vi "Get Access Mode.vi"(8 "error in (no error)":errorcluster, 11 "Process In":refnum<class "Process.lvclass">) -> (0 "error out":errorcluster, 2 "Access Mode":T1, 3 "Process Out":refnum<class "Process.lvclass">)   [LabVIEW 2020, in "Process.lvclass"]
doc: "Get the recommended access mode for accessing the class attributes. Request means that a request should be made to the running process and Read means that the data should be read directly from the attributes."
uses:
  Process.lvclass
  TypeDefs/Access Mode.ctl
  Process.lvclass/Process.ctl
  <vilib>/Utility/error.llb/Clear Errors.vi
  <vilib>/Utility/error.llb/Error Cluster From Error Code.vi
  <vilib>/ErrorRing/Error Ring.xnode
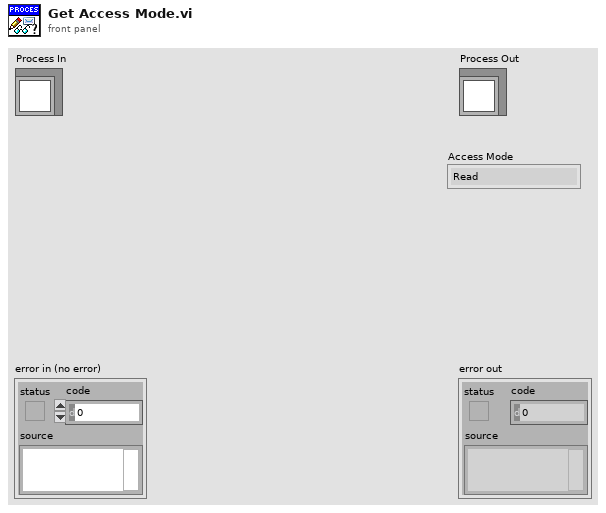
[diagram p1: front panel]
types:
  T1 = typedef "Process.lvclass/Access Mode.ctl" = enum16{"Read", "Request"}
  T2 = typedef "Process.lvclass/Lifecycle State.ctl" = enum16{"Uninitialized", "Initialized", "Started", "Running", "Stopped", "Finished"}
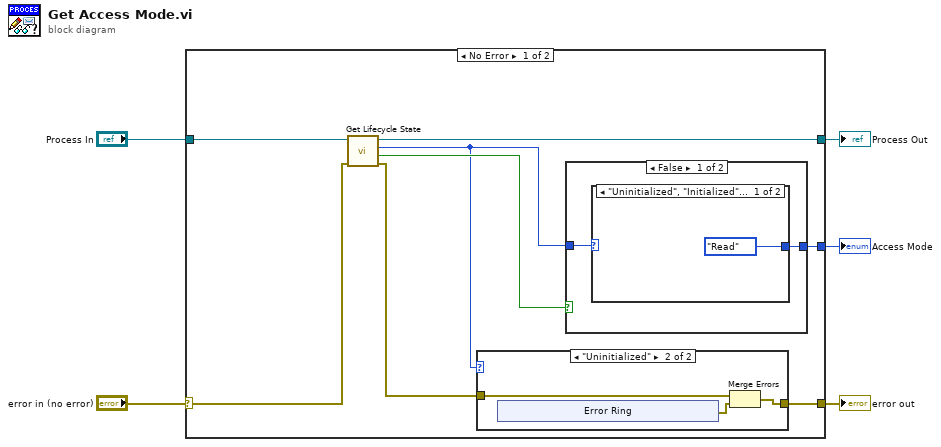
[diagram p0: block diagram]
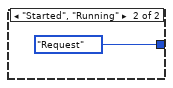
[diagram p3: hidden frame]
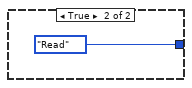
[diagram p4: hidden frame]
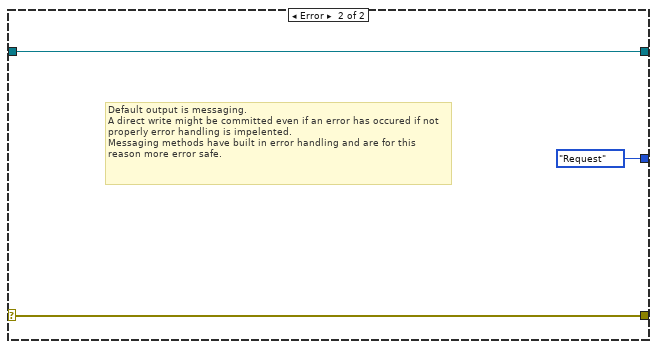
[diagram p5: hidden frame]
diagram:
  n1 = case shown="No Error" "error in (no error)" {
    selector: "error in (no error)" -> [w11 w27]
    tunnel: "Process In" -> [w13 w29]
    tunnel: [w12 w29] -> w4
    tunnel: [w7 w27] -> w2
    tunnel: [w9 Access_Mode."Request" ("Access Mode")] -> w1
    frame No Error {
      n2 = call "Get Lifecycle State.vi"("error in (no error)"=w11, "Process In"=w13) -> ("error out"=w6:errorcluster, "In Process Loop?"=w10:bool, "Lifecycle State"=w8:T2, "Process Out"=w12:refnum<class "Process.lvclass">)  [unwired: 6 in]
      n3 = case shown="\"Uninitialized\"" w8 {
        tunnel: [w14 w16] -> w7
        tunnel: w6 -> [w14 w15]
        frame Default {
        }
        frame "Uninitialized" {
          n4 = xnode "Error Ring"() -> ("error out"=w17:errorcluster)
          n5 = Merge Errors(w15, w17) -> (w16:errorcluster)
        }
      }
      n6 = case shown="False" w10 {
        tunnel: w8 -> [w23 _]
        tunnel: [w22 Access_Mode."Read" ("Access Mode")] -> w9
        frame False {
          n7 = case shown="\"Uninitialized\", \"Initialized\", \"Stopped\", \"Finished\"" w23 {
            tunnel: [Access_Mode."Read" ("Access Mode") Access_Mode."Request" ("Access Mode")] -> w22
            frame "Uninitialized", "Initialized", "Stopped", "Finished" {
            }
            frame "Started", "Running" {
            }
          }
        }
        frame True {
        }
      }
    }
    frame Error {
      # "Default output is messaging. \nA direct write might be committed even if an error has occured if not properly error handling is impelented.\nMessaging methods have built in error handling and are for this reason more error safe."
    }
  }
  "error out" <- w2
  "Process Out" <- w4
  "Access Mode" <- w1
